vi "FolderMon Daemon.vi"() -> ()   [LabVIEW 2011]
uses:
  FolderMon events.ctl
  FolderMon config.ctl
  server lib/Spartan CONFIG Global.vi
  server lib/Spartan Version.vi
panel:
  in  "Monitoring":T1[](array[typedef])
  out "FolderMon":refnum<user-event>
  in  "start":T2
  in  "Polling":i32=10000
  # "Don't change the control/indicator names\nas they're used through VI server...."
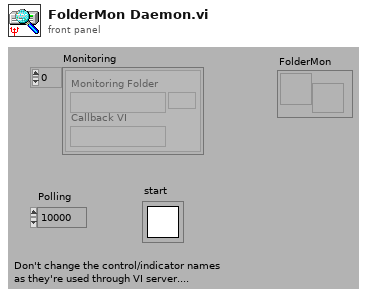
[diagram p1: front panel]
types:
  T1 = typedef "FolderMon config.ctl" = cluster{"Monitoring Folder":path, "Callback VI":string}
  T2 = typedef "Rendezvous RefNum" = refnum<k1>
  T3 = typedef "FolderMon events.ctl" = enum16{"stop", "update"}
  T4 = typedef "Keyed Array.ctl" = cluster{"keys":string[], "values":string[]}
  T5 = typedef "FolderMon changes.ctl" = enum16{"None", "First", "New", "Properties", "Deleted"}
  T6 = cluster{"Folder":path, "Changed Files":cluster{string, "Change":T5}[]}
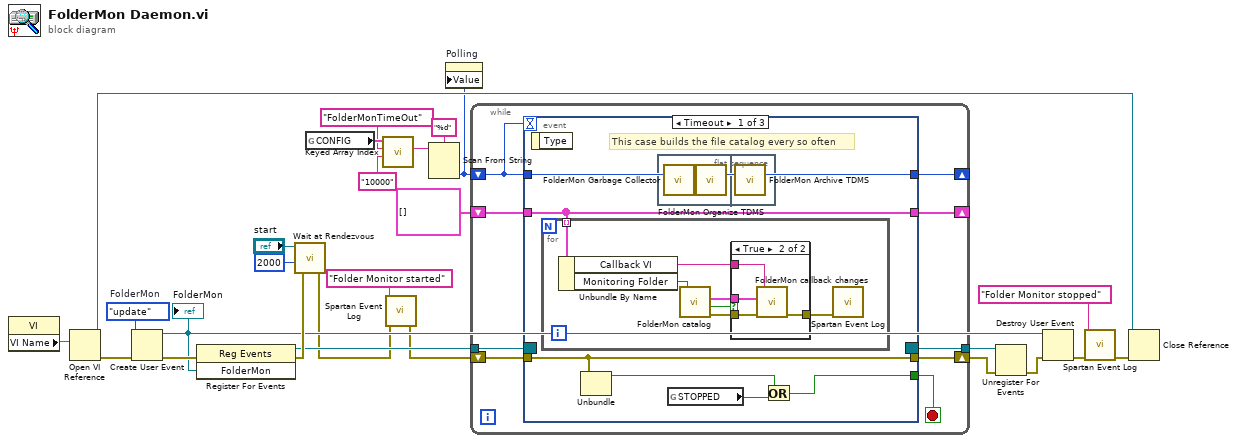
[diagram p0: block diagram]
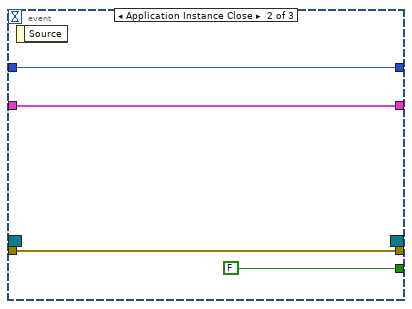
[diagram p3: hidden frame]
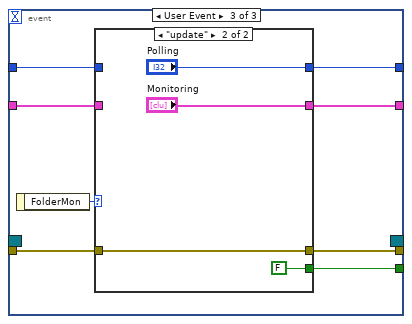
[diagram p4: hidden frame]
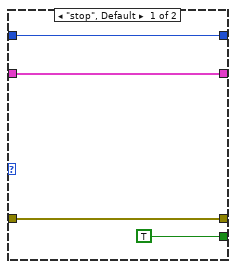
[diagram p5: hidden frame]
diagram:
  w14 = FolderMon_events."update"  # FolderMon
  n1 = property class="VI"() -> ("VI Name"=w23:string)  [unwired: 2 in, 2 out]
  n2 = Open VI Reference(vi path=w23) -> (vi reference=w24:refnum<vi>, error out=w22:errorcluster)  [unwired: 1 in, 4 out]
  n3 = Create User Event(user event datatype=w14, error in=w22) -> (user event=w15:refnum<user-event>, error out=w21:errorcluster)
  "FolderMon" <- w15
  n4 = register-events(error in=w21, w15) -> (reference out=w16:refnum<event-registration>, error out=w20:errorcluster)  [unwired: 1 in]
  n5 = call <vilib>:"Wait at Rendezvous.vi"("error in (no error)"=w20, "ms timeout (-1)"=2000, "rendezvous"="start") -> ("error out"=w9:errorcluster)  [unwired: 4 out]
  n6 = global read "Spartan CONFIG Global.vi" "CONFIG"() -> (w6:T4)
  n7 = call "Keyed Array Index.vi"("default value"="10000", "key"="FolderMonTimeOut", "array in"=w6) -> ("value"=w3:string)  [unwired: 1 in, 3 out]
  n8 = call "Spartan Event Log.vi"("error in (no error)"=w9, "message (\"\")"="Folder Monitor started" ("name (unnamed)")) -> ("error out"=w8:errorcluster)  [unwired: 3 in, 3 out]
  n9 = Scan From String(format string="%d", input string=w3) -> (output 1=w1:i32)  [unwired: 3 in, 3 out]
  n10 = property on="Polling" class="DigNum (strict)"("Value"=w1) -> ()  [unwired: 2 in, 2 out]
  n11 = while {
    shift-right: [w35] -> _
    shift-left: w1 -> [w34]
    shift-right: [w32] -> _
    shift-left: T1[] [] -> [w33]
    shift-right: [w30] -> w18
    shift-left: w8 -> [w31]
    tunnel: w16 -> [w28]
    tunnel: [w27] -> w19
    stop <- w29 stop-if-true
    n12 = event shown="[0] Timeout" {
      selector: w28 -> [_ _ _]
      dyn-events: [_ _ _] -> w27
      timeout: w34 -> [_ _ _]
      tunnel: [w40 w57 w59] -> w35
      tunnel: w34 -> [w40 w57 w62]
      tunnel: w33 -> [w36 w56 w61]
      tunnel: [w36 w56 w60] -> w32
      tunnel: w31 -> [w41 w54 w64]
      tunnel: [w41 w54 w63] -> w30
      tunnel: [w37 FALSE w58] -> w29
      event Timeout {
        # "This case builds the file catalog every so often"
        n13 = event-data() -> ()  [unwired: 2 out]
        n14 = for {
          tunnel: w36 -> [w48] mode=indexing
          n15 = Unbundle By Name(w48) -> ("Callback VI"=w45:string, "Monitoring Folder"=w44:path)
          n16 = call "FolderMon catalog.vi"("Folder"=w44) -> ("error out"=w47:errorcluster, "Any Changes?"=w43:bool, "Changes"=w42:T6)  [unwired: 1 in, 3 out]
          n17 = case shown="True" w43 {
            tunnel: w47 -> [w49 w53]
            tunnel: [w49 w52] -> w46
            tunnel: w45 -> [_ w51]
            tunnel: w42 -> [_ w50]
            frame False {
            }
            frame True {
              n18 = call "FolderMon callback changes.vi"("error in (no error)"=w53, "Changes"=w50, "Callback VI Name (Empty)"=w51) -> ("error out"=w52:errorcluster)  [unwired: 4 out]
            }
          }
          n19 = call "Spartan Event Log.vi"("error in (no error)"=w46) -> ()  [unwired: 4 in, 4 out]
        }
        n20 = Unbundle(w41) -> ("status"=w38:bool)  [unwired: 2 out]
        n21 = flat-sequence {
          frame #0 {
            n22 = call "FolderMon Garbage Collector.vi"() -> ()  [unwired: 1 out]
            n23 = call "FolderMon Organize TDMS.vi"() -> ()  [unwired: 1 in]
          }
          frame #1 {
            n24 = call "FolderMon Archive TDMS.vi"() -> ()  [unwired: 1 in]
          }
        }
        n25 = global read "Spartan Version.vi" "STOPPED"() -> (w39:bool)
        n26 = Or(x=w38, y=w39) -> (x .or. y?=w37:bool)
      }
      event Application Instance Close {
        n27 = event-data() -> ()  [unwired: 2 out]
      }
      event User Event {
        n28 = event-data() -> ("FolderMon"=w65:T3)  [unwired: 1 out]
        n29 = case shown="\"update\"" w65 {
          tunnel: w64 -> [w69 w72]
          tunnel: [w69 w72] -> w63
          tunnel: w62 -> [w67 _]
          tunnel: w61 -> [w68 _]
          tunnel: [w68 "Monitoring"] -> w60
          tunnel: [w67 "Polling"] -> w59
          tunnel: [TRUE FALSE] -> w58
          frame "stop", Default {
          }
          frame "update" {
          }
        }
      }
    }
  }
  n30 = Unregister For Events(event registration refnum=w19, error in=w18) -> (error out=w17:errorcluster)
  n31 = Destroy User Event(user event=w15, error in=w17) -> (error out=w11:errorcluster)
  n32 = call "Spartan Event Log.vi"("error in (no error)"=w11, "message (\"\")"="Folder Monitor stopped" ("name (unnamed)")) -> ("error out"=w10:errorcluster)  [unwired: 3 in, 3 out]
  n33 = Close Reference(reference=w24, error in (no error)=w10) -> ()  [unwired: 1 out]
